vi "简易跑马灯.vi"() -> ()   [LabVIEW 2013]
panel:
  out "Lamp":bool[](array[boolean])
  in  "延时时间 (s)":dbl=1.0 caption="目标时间(s)"
  in  "停止":bool
  in  "Num":i32
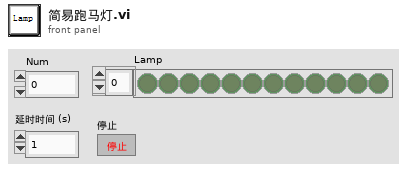
[diagram p1: front panel]
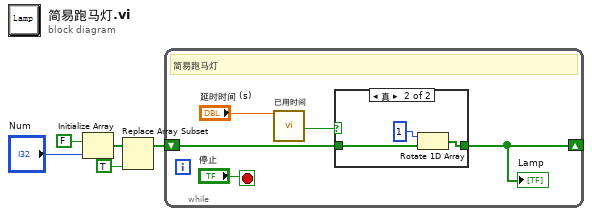
[diagram p0: block diagram]
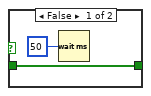
[diagram p2: hidden frame]
diagram:
  n1 = Initialize Array(FALSE, "Num") -> (w3:bool[])
  n2 = Replace Array Subset(array=w3, new element=TRUE ("新元素/子数组")) -> (w1:bool[])  [unwired: 1 in]
  n3 = while {
    shift-right: [w8] -> _
    shift-left: w1 -> [w9]
    stop <- "停止" stop-if-true
    # "简易跑马灯"
    n4 = call "已用时间"("Time Target (s)"="延时时间 (s)") -> ("Time has Elapsed"=w6:bool)  [unwired: 11 in, 7 out]
    n5 = case shown="真" w6 {
      tunnel: w9 -> [w12 w15]
      tunnel: [w12 w13] -> w8
      frame False {
        n6 = Wait (ms)(milliseconds to wait=u32 50 ("等待时间（毫秒）")) -> ()  [unwired: 1 out]
      }
      frame True {
        n7 = Rotate 1D Array(1:w15, 2:1 ("n")) -> (0:w13:bool[])
      }
    }
    "Lamp" <- w8
  }
